vi "GetTxStatus.vi"(6 "Legacy (f)?":bool, 8 "error in (no error)":errorcluster) -> (0 "error out":errorcluster, 2 "Tx Stat":T1)   [LabVIEW 2011]
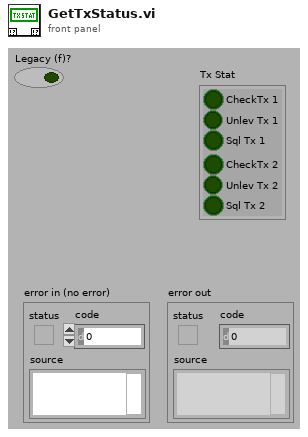
[diagram p1: front panel]
types:
  T1 = cluster{"CheckTx 1":bool, "Unlev Tx 1":bool, "Sql Tx 1":bool, "CheckTx 2":bool, "Unlev Tx 2":bool, "Sql Tx 2":bool}
  T2 = cluster{"Boolean out[0]":bool, "Boolean out[1]":bool, "Boolean out[2]":bool, "Boolean out[3]":bool, "Boolean out[4]":bool, "Boolean out[5]":bool}
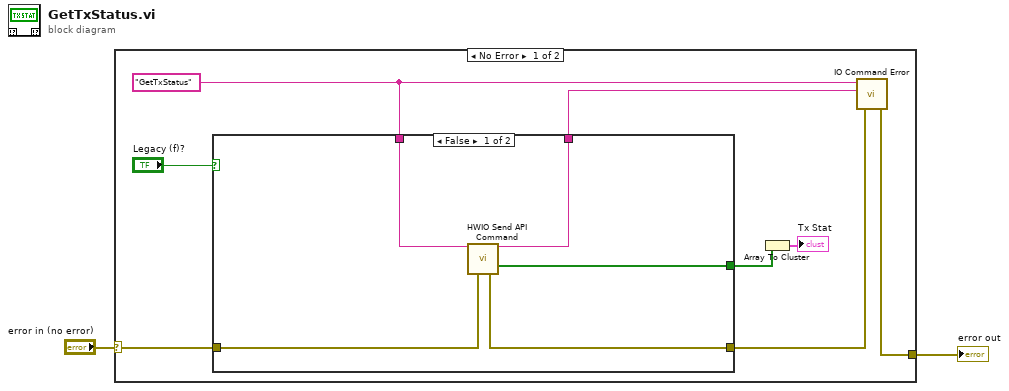
[diagram p0: block diagram]
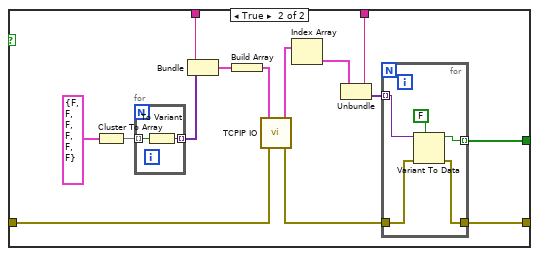
[diagram p2: hidden frame]
diagram:
  n1 = case shown="No Error" "error in (no error)" {
    selector: "error in (no error)" -> [w3 w37]
    tunnel: [w7 w37] -> w2
    frame No Error {
      w6 = "GetTxStatus"
      n2 = case shown="False" "Legacy (f)?" {
        tunnel: [w13 w24] -> w10
        tunnel: w3 -> [w15 w22]
        tunnel: [w14 w21] -> w8
        tunnel: w6 -> [w11 w20]
        tunnel: [w12 w19] -> w5
        frame False {
          n3 = call "HWIO Send API Command.vi"("Action"=w11, "error in (no error)"=w15) -> ("Action out"=w12:string, "Boolean out"=w13:bool[], "error out"=w14:errorcluster)  [unwired: 6 in, 5 out]
        }
        frame True {
          n4 = Cluster To Array(cluster=T1 {"CheckTx 1"=FALSE, "Unlev Tx 1"=FALSE, "Sql Tx 1"=FALSE, "CheckTx 2"=FALSE, "Unlev Tx 2"=FALSE, "Sql Tx 2"=FALSE} ("Tx Stat")) -> (array=w26:bool[])
          n5 = for {
            tunnel: w26 -> [w31] mode=indexing
            tunnel: [w30] -> w25 mode=indexing
            n6 = To Variant(anything=w31) -> (Variant=w30:variant)
          }
          n7 = Bundle(w20, w25) -> (w29:cluster{string, variant[]})  [unwired: 1 out]
          n8 = Build Array(w29) -> (w16:cluster{string, variant[]}[])
          n9 = call "TCPIP IO.vi"("error in (no error)"=w22, "Commands"=w16) -> ("error out"=w23:errorcluster, "Responses"=w18:cluster{string, variant[]}[])  [unwired: 1 in, 3 out]
          n10 = Index Array(array=w18) -> (element=w17:cluster{string, variant[]})  [unwired: 1 in]
          n11 = Unbundle(w17) -> (w19:string, w28:variant[])
          n12 = for {
            tunnel: [w36] -> w21
            tunnel: [w35] -> w24 mode=indexing
            tunnel: w23 -> [w34]
            tunnel: w28 -> [w33] mode=indexing
            n13 = Variant To Data(error in=w34, type=FALSE, Variant=w33) -> (data=w35:bool, error out=w36:errorcluster)
          }
        }
      }
      n14 = Array To Cluster(array=w10) -> (cluster=→"Tx Stat":T2)
      n15 = call "IO Command Error.vi"("error in (no error)"=w8, "Command Returned (\"\")"=w5, "Command Sent (\"\")"=w6) -> ("error out"=w7:errorcluster)  [unwired: 4 out]
    }
    frame Error {
    }
  }
  "error out" <- w2
